vi "Spike Kicker.vi"   [LabVIEW 2012]
uses:
  <vilib>/Rock Robotics/WPI/Relay/WPI_RelayValue.ctl
  <vilib>/Rock Robotics/WPI/Joystick/WPI_JoystickGetSetRefNum.vi
  Globals/Useful Values.vi
types:
  T1 = typedef "WPI_RelayValue.ctl" = enum16{"Off", "On", "Forward", "Reverse"}
  T2 = typedef "WPI_JoystickDevRef.ctl" = cluster{"Device":T3}
  T3 = typedef "WPI_JoystickDeviceEnum.ctl" = enum16{"USB 1", "USB 2", "USB 3", "USB 4", "Kinect 1", "Kinect 2"}
  T4 = typedef "WPI_DigitalInputDevRef.ctl" = cluster{"DevStatus":errorcluster, "DIO Channel":T5, "Digital Module":T6}
  T5 = typedef "FPGA_DIOChannel.ctl" = enum8{"DIO 1", "DIO 2", "DIO 3", "DIO 4", "DIO 5", "DIO 6", "DIO 7", "DIO 8", "DIO 9", "DIO 10", "DIO 11", "DIO 12", "DIO 13", "DIO 14", "Invalid"}
  T6 = typedef "FPGA_TypedefDigitalModule.ctl" = enum16{"Digital Module 1", "Digital Module 2"}
  T7 = typedef "WPI_RelayDevRef.ctl" = cluster{"DevStatus":errorcluster, "Relay Channel":T8, "Digital Module":T6, "Relay Direction":T9}
  T8 = typedef "FPGA_DIORelayChannel.ctl" = enum8{"Relay 1", "Relay 2", "Relay 3", "Relay 4", "Relay 5", "Relay 6", "Relay 7", "Relay 8", "Invalid"}
  T9 = typedef "WPI_RelayDirection.ctl" = enum16{"Both directions", "Forward only", "Reverse only"}
  T10 = typedef "WPI_JoystickButtonState.ctl" = cluster{"Button 1":bool, "Button 2":bool, "Button 3":bool, "Button 4":bool, "Button 5":bool, "Button 6":bool, "Button 7":bool, "Button 8":bool, "Button 9":bool, "Button 10":bool, "Button 11":bool, "Button 12":bool}
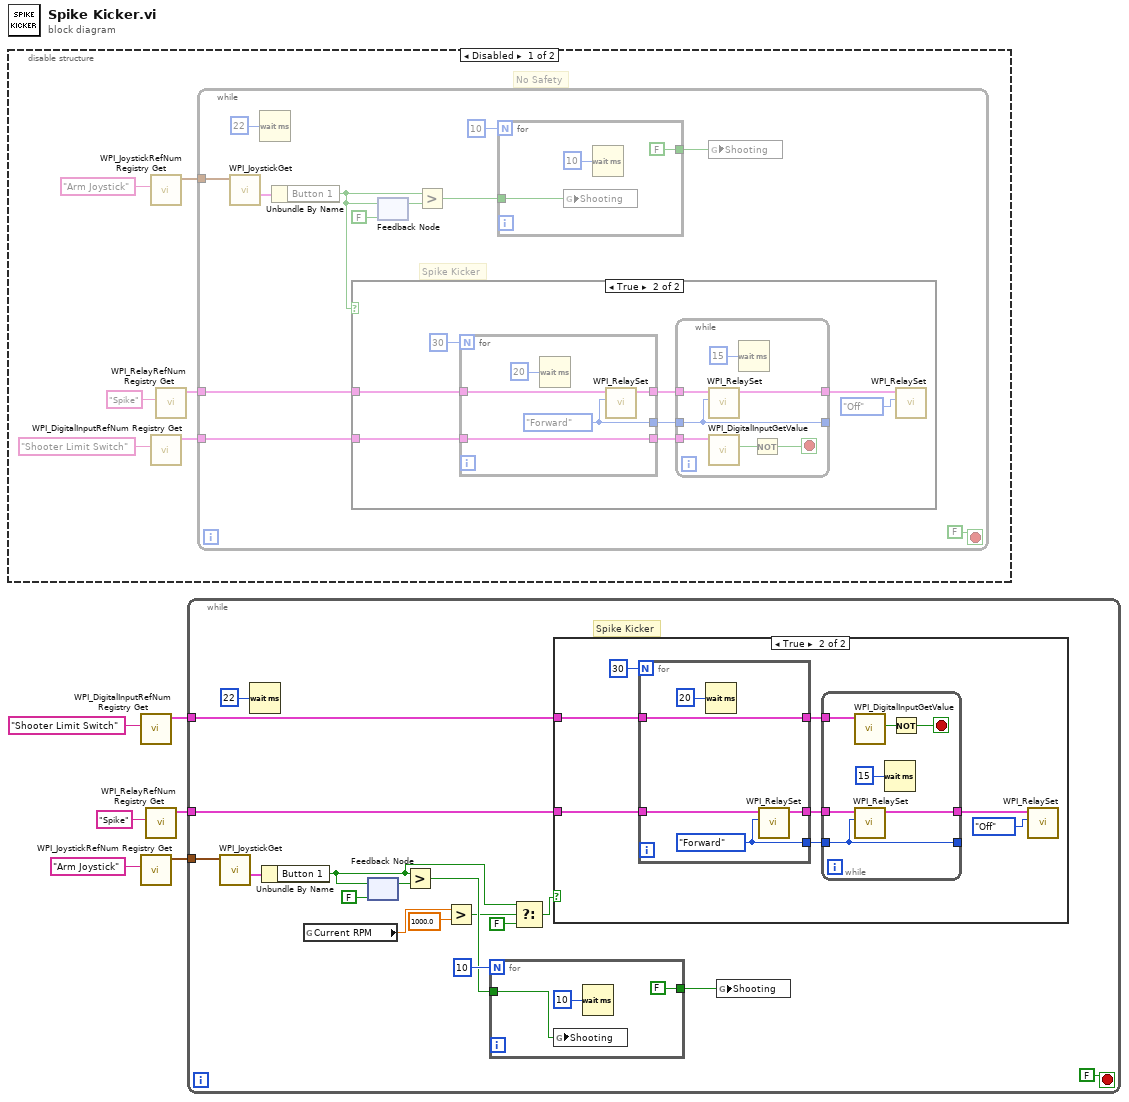
[diagram p0: block diagram]
diagram:
  n1 = disable-structure shown="Disabled" {
    frame Disabled {
      # "No Safety"
      n2 = call <vilib>:"WPI_JoystickRefNum Registry Get.vi"("refnum name"="Arm Joystick") -> ("JoystickDevRef"=w8:T2)  [unwired: 9 in, 1 out]
      n3 = call <vilib>:"WPI_DigitalInputRefNum Registry Get.vi"("refnum name"="Shooter Limit Switch") -> ("DigitalInputDevRef"=w10:T4)  [unwired: 9 in, 1 out]
      n4 = call <vilib>:"WPI_RelayRefNum Registry Get.vi"("refnum name"="Spike") -> ("RelayDevRef"=w11:T7)  [unwired: 9 in, 1 out]
      n5 = while {
        tunnel: w8 -> [w23]
        tunnel: w11 -> [w19]
        tunnel: w10 -> [w20]
        stop <- FALSE stop-if-true
        # "Spike Kicker"
        n6 = call <vilib>:"WPI_JoystickGet.vi"("JoystickDevRef"=w23) -> ("Buttons"=w22:T10)  [unwired: 1 in, 5 out]
        n7 = Wait (ms)(milliseconds to wait=u32 22) -> ()  [unwired: 1 out]
        n8 = Unbundle By Name(w22) -> ("Button 1"=w16:bool)
        n9 = case shown="True" w16 {
          tunnel: w19 -> [_ w35]
          tunnel: w20 -> [_ w30]
          frame False {
          }
          frame True {
            n10 = for {
              N: 30 -> [_]
              tunnel: w35 -> [w46]
              tunnel: [w45] -> w33
              tunnel: [w44] -> w32
              tunnel: [w43] -> w31
              tunnel: w30 -> [w43]
              w44 = WPI_RelayValue."Forward" ("RelayValue")
              n11 = Wait (ms)(milliseconds to wait=u32 20) -> ()  [unwired: 1 out]
              n12 = call <vilib>:"WPI_RelaySet.vi"("RelayValue"=w44, "RelayDevRef"=w46) -> ("RelayDevRef"=w45:T7)  [unwired: 8 in, 1 out]
            }
            n13 = while {
              tunnel: w33 -> [w42]
              tunnel: [w40] -> w29
              tunnel: [w38] -> _
              tunnel: w32 -> [w38]
              tunnel: w31 -> [w37]
              stop <- w36 stop-if-true
              n14 = call <vilib>:"WPI_RelaySet.vi"("RelayValue"=w38, "RelayDevRef"=w42) -> ("RelayDevRef"=w40:T7)  [unwired: 8 in, 1 out]
              n15 = call <vilib>:"WPI_DigitalInputGetValue.vi"("DigitalInputDevRef"=w37) -> ("Value"=w39:bool)  [unwired: 8 in, 2 out]
              n16 = Wait (ms)(milliseconds to wait=u32 15) -> ()  [unwired: 1 out]
              n17 = Not(x=w39) -> (.not. x?=w36:bool)
            }
            n18 = call <vilib>:"WPI_RelaySet.vi"("RelayValue"=WPI_RelayValue."Off", "RelayDevRef"=w29) -> ()  [unwired: 8 in, 2 out]
          }
        }
        n19 = feedback-in #1(w16) -> ()
        n20 = feedback #1(FALSE ("Button 1")) -> (w17:bool)
        n21 = Greater?(x=w16, y=w17) -> (0:w14:bool)
        n22 = for {
          N: 10 -> [_]
          tunnel: w14 -> [w27]
          tunnel: [FALSE ("Shooting")] -> w13
          n23 = global write "Useful Values.vi" "Shooting"(w27) -> ()
          n24 = Wait (ms)(milliseconds to wait=u32 10) -> ()  [unwired: 1 out]
        }
        n25 = global write "Useful Values.vi" "Shooting"(w13) -> ()
      }
    }
    frame Enabled {
    }
  }
  n26 = call <vilib>:"WPI_DigitalInputRefNum Registry Get.vi"("refnum name"="Shooter Limit Switch") -> ("DigitalInputDevRef"=w3:T4)  [unwired: 9 in, 1 out]
  n27 = call <vilib>:"WPI_JoystickRefNum Registry Get.vi"("refnum name"="Arm Joystick") -> ("JoystickDevRef"=w5:T2)  [unwired: 9 in, 1 out]
  n28 = call <vilib>:"WPI_RelayRefNum Registry Get.vi"("refnum name"="Spike") -> ("RelayDevRef"=w2:T7)  [unwired: 9 in, 1 out]
  n29 = while {
    tunnel: w5 -> [w63]
    tunnel: w2 -> [w59]
    tunnel: w3 -> [w60]
    stop <- FALSE stop-if-true
    # "Spike Kicker"
    n30 = call <vilib>:"WPI_JoystickGet.vi"("JoystickDevRef"=w63) -> ("Buttons"=w62:T10)  [unwired: 1 in, 5 out]
    n31 = Wait (ms)(milliseconds to wait=u32 22) -> ()  [unwired: 1 out]
    n32 = Unbundle By Name(w62) -> ("Button 1"=w52:bool)
    n33 = global read "Useful Values.vi" "Current RPM"() -> (w50:dbl)
    n34 = feedback-in #2(w52) -> ()
    n35 = feedback #2(FALSE ("Button 1")) -> (w57:bool)
    n36 = Greater?(x=w52, y=w57) -> (0:w55:bool)
    n37 = Greater?(x=w50, y=1000.0) -> (0:w48:bool)
    n38 = for {
      N: 10 -> [_]
      tunnel: w55 -> [w67]
      tunnel: [FALSE ("Shooting")] -> w54
      n39 = global write "Useful Values.vi" "Shooting"(w67) -> ()
      n40 = Wait (ms)(milliseconds to wait=u32 10) -> ()  [unwired: 1 out]
    }
    n41 = Select(t=w52, s=w48, f=FALSE ("Button 1")) -> (s? t:f=w51:bool)
    n42 = case shown="True" w51 {
      tunnel: w59 -> [_ w75]
      tunnel: w60 -> [_ w70]
      frame False {
      }
      frame True {
        n43 = for {
          N: 30 -> [_]
          tunnel: w75 -> [w86]
          tunnel: [w85] -> w73
          tunnel: [w84] -> w72
          tunnel: [w83] -> w71
          tunnel: w70 -> [w83]
          w84 = WPI_RelayValue."Forward" ("RelayValue")
          n44 = Wait (ms)(milliseconds to wait=u32 20) -> ()  [unwired: 1 out]
          n45 = call <vilib>:"WPI_RelaySet.vi"("RelayValue"=w84, "RelayDevRef"=w86) -> ("RelayDevRef"=w85:T7)  [unwired: 8 in, 1 out]
        }
        n46 = while {
          tunnel: w73 -> [w82]
          tunnel: [w80] -> w69
          tunnel: [w78] -> _
          tunnel: w72 -> [w78]
          tunnel: w71 -> [w77]
          stop <- w76 stop-if-true
          n47 = call <vilib>:"WPI_DigitalInputGetValue.vi"("DigitalInputDevRef"=w77) -> ("Value"=w79:bool)  [unwired: 8 in, 2 out]
          n48 = call <vilib>:"WPI_RelaySet.vi"("RelayValue"=w78, "RelayDevRef"=w82) -> ("RelayDevRef"=w80:T7)  [unwired: 8 in, 1 out]
          n49 = Wait (ms)(milliseconds to wait=u32 15) -> ()  [unwired: 1 out]
          n50 = Not(x=w79) -> (.not. x?=w76:bool)
        }
        n51 = call <vilib>:"WPI_RelaySet.vi"("RelayValue"=WPI_RelayValue."Off", "RelayDevRef"=w69) -> ()  [unwired: 8 in, 2 out]
      }
    }
    n52 = global write "Useful Values.vi" "Shooting"(w54) -> ()
  }
